vi "FIFO_type.vi"() -> ()   [LabVIEW 2017]
panel:
  in  "Numeric":i16
  in  "Boolean":bool
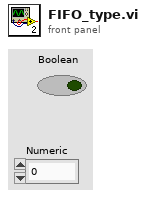
[diagram p1: front panel]
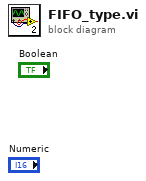
[diagram p0: block diagram]
diagram:
